vi "ComputeAnnulusROIArray.vi"(7 "ROIDim":T2, 8 "error in (no error)":errorcluster, 10 "ROI In":T1 {"Contours"."Type" items=["No Selection", "Point", "Line", "Rectangle", "Oval", "Polygon", "Freehand Region", "Annulus", "Unused2", "Unused3", "Broken Line", "Freehand Line", "Rotated Rectangle"]}) -> (0 "error out":errorcluster, 2 "ROIArray":T1[](array[typedef]) {"Contours"."Type" items=["No Selection", "Point", "Line", "Rectangle", "Oval", "Polygon", "Freehand Region", "Annulus", "Unused2", "Unused3", "Broken Line", "Freehand Line", "Rotated Rectangle"]})   [LabVIEW 2019]
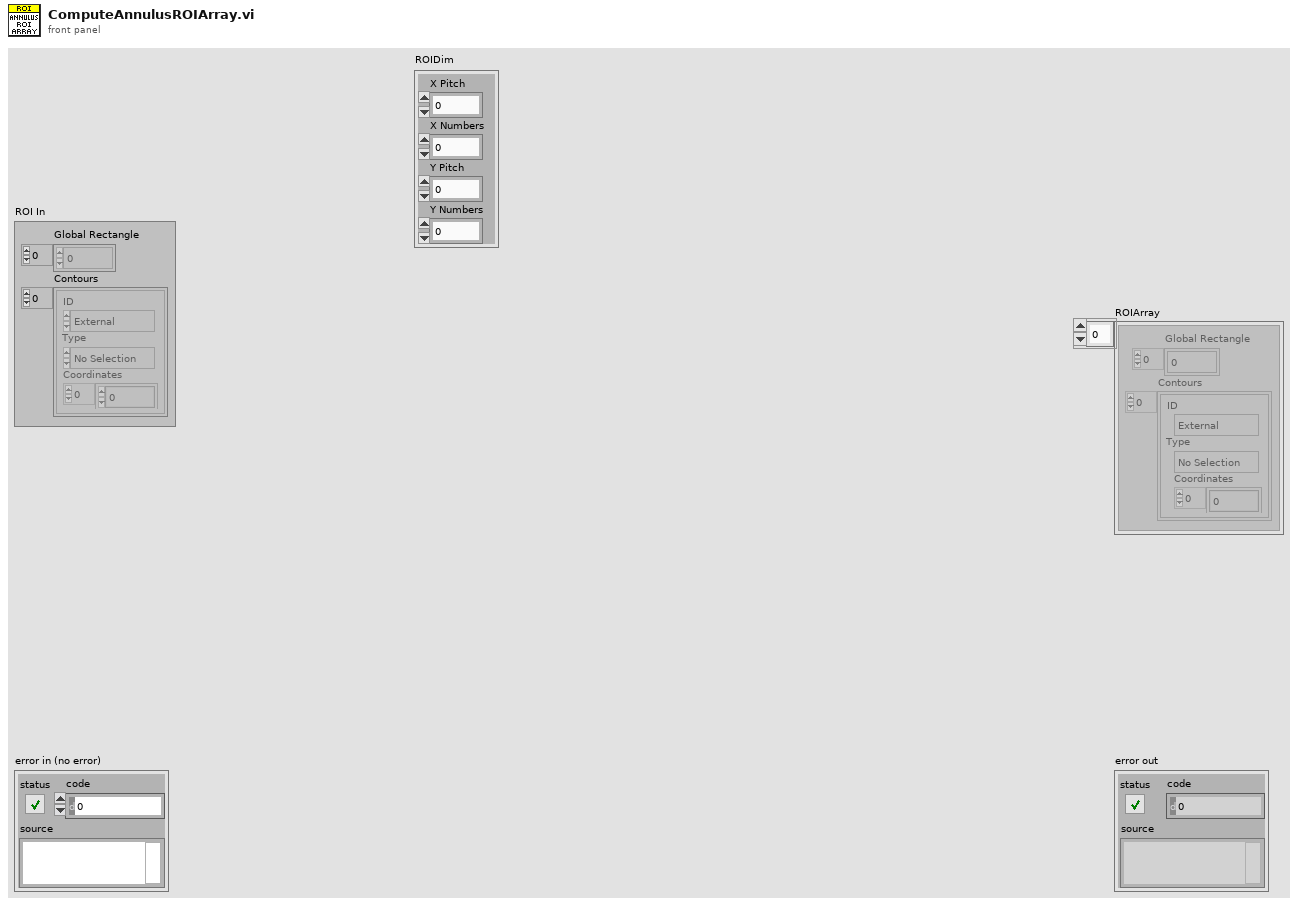
[diagram p1: front panel]
types:
  T1 = typedef "ROI Descriptor" = cluster{"Global Rectangle":i32[], "Contours":cluster{"ID":enum32{"External", "Internal"}, "Type":u32, "Coordinates":i32[]}[]}
  T2 = cluster{"X Pitch":i32, "X Numbers":i32, "Y Pitch":i32, "Y Numbers":i32}
  T3 = typedef "IMAQ Circle" = cluster{"Center X":i32, "Center Y":i32, "Inner Radius":i32, "Outer Radius":i32, "Start Angle":dbl, "End Angle":dbl}
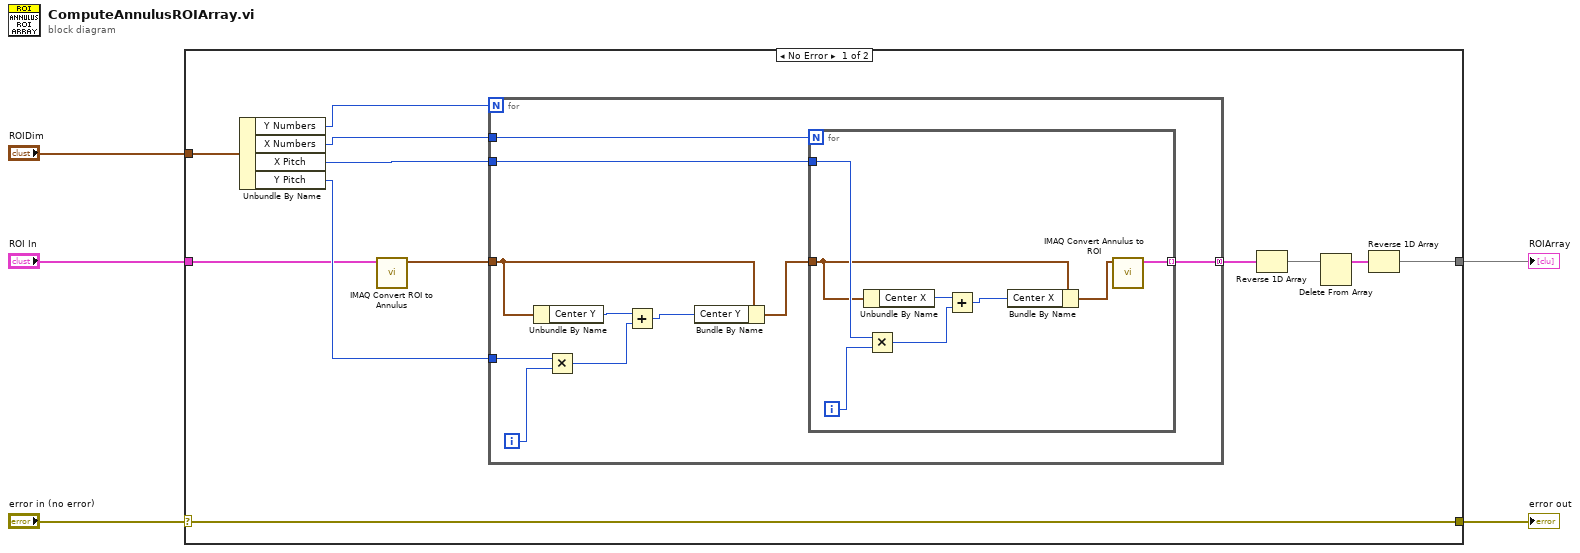
[diagram p0: block diagram]
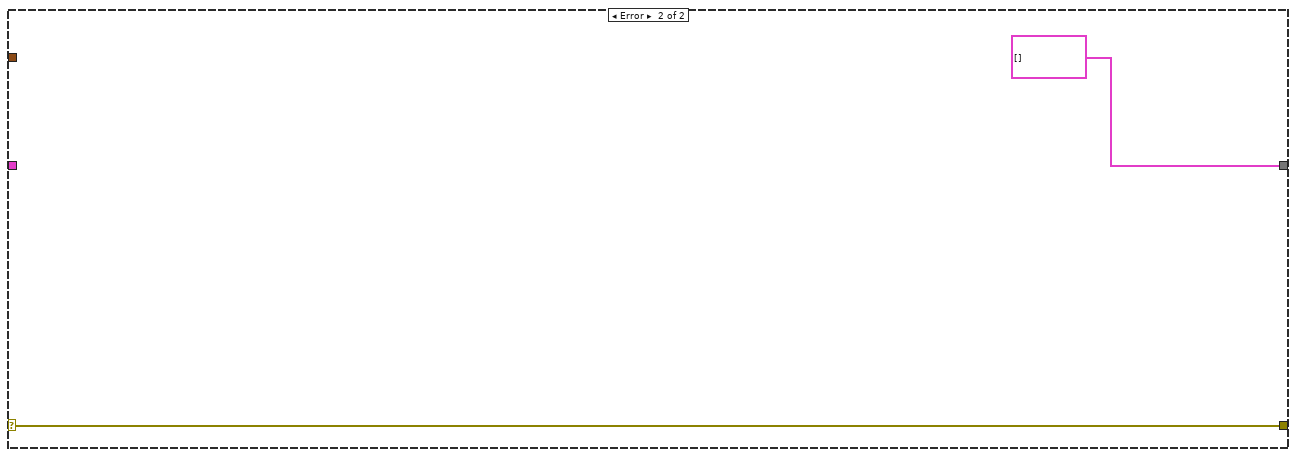
[diagram p2: hidden frame]
diagram:
  n1 = case shown="No Error" "error in (no error)" {
    selector: "error in (no error)" -> [w11 w37]
    tunnel: "ROIDim" -> [w17 _]
    tunnel: [w6 T1[] []] -> w4
    tunnel: [w11 w37] -> w2
    tunnel: "ROI In" -> [w8 _]
    frame No Error {
      n2 = Unbundle By Name(w17) -> ("Y Numbers"=w16:i32, "X Numbers"=w15:i32, "X Pitch"=w13:i32, "Y Pitch"=w14:i32)
      n3 = call "IMAQ Convert ROI to Annulus"("ROI Descriptor"=w8) -> ("Annulus"=w9:T3)  [unwired: 8 in, 1 out]
      n4 = for {
        N: w16 -> [_]
        tunnel: w15 -> [w27]
        tunnel: w9 -> [w21]
        tunnel: w14 -> [w22]
        tunnel: w13 -> [w19]
        tunnel: [w18] -> w12 mode=concatenating
        i -> [w23]
        n5 = Unbundle By Name(w21) -> ("Center Y"=w24:i32)
        n6 = Multiply(x=w22, y=w23) -> (x*y=w26:i32)
        n7 = Add(x=w24, y=w26) -> (x+y=w25:i32)
        n8 = Bundle By Name(cluster=w21, "Center Y"=w25) -> (w20:T3)
        n9 = for {
          N: w27 -> [_]
          tunnel: w20 -> [w30]
          tunnel: w19 -> [w32]
          tunnel: [w28] -> w18 mode=indexing
          i -> [w29]
          n10 = Unbundle By Name(w30) -> ("Center X"=w35:i32)
          n11 = Multiply(x=w32, y=w29) -> (x*y=w33:i32)
          n12 = Add(x=w35, y=w33) -> (x+y=w34:i32)
          n13 = Bundle By Name(cluster=w30, "Center X"=w34) -> (w31:T3)
          n14 = call "IMAQ Convert Annulus to ROI"("Annulus"=w31) -> ("ROI Descriptor"=w28:T1)  [unwired: 8 in, 1 out]
        }
      }
      n15 = Reverse 1D Array(array=w12) -> (reversed array=w7:T1[])
      n16 = Delete From Array(array=w7) -> (array with subset deleted=w10:T1[])  [unwired: 2 in, 1 out]
      n17 = Reverse 1D Array(array=w10) -> (reversed array=w6:T1[])
    }
    frame Error {
    }
  }
  "ROIArray" <- w4
  "error out" <- w2
